vi "AdaptToInputs.vi"(0 "XRef":T8, 1 "Term Types":T5, 2 "State In":T1={"Type"=variant(bool FALSE)}) -> (14 "Reply":T3, 15 "Fatal Error Out":T2, 16 "State Out":T1={"Type"=variant(bool FALSE)})   [LabVIEW 2014, in "TagDB(dev).lvlib" / "tagDB_setValue.xnode"]
uses:
  tagDB_setValue.xnode
  <vilib>/XNodeSupport/XNodeXNodeRef.ctl
  <vilib>/XNodeSupport/XNodeTermTypeIDPairs.ctl
  <vilib>/XNodeSupport/XNodeTermTypeIDPair.ctl
  <vilib>/XNodeSupport/XNodeType.ctl
  <vilib>/XNodeSupport/XNodeString.ctl
  State.ctl
  <vilib>/XNodeSupport/XNodeStringArray.ctl
  <vilib>/XNodeSupport/XNodeErrorCluster.ctl
  <vilib>/XNodeSupport/NI_XNodeSupport.lvlib
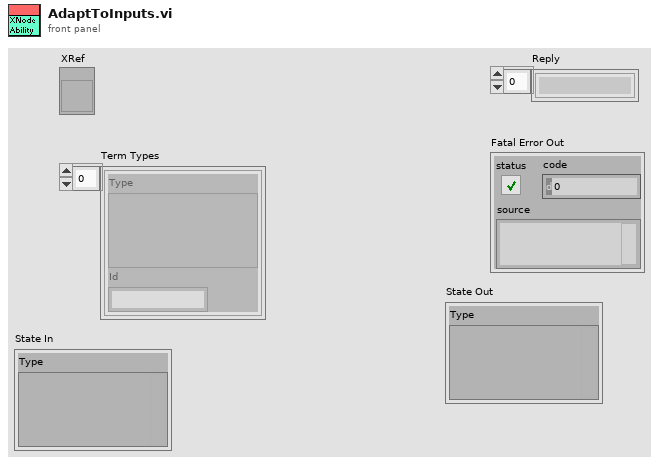
[diagram p1: front panel]
types:
  T1 = typedef "TagDB(dev).lvlib/tagDB_setValue.xnode/State.ctl" = cluster{"Type":variant}
  T2 = typedef "NI_XNodeSupport.lvlib/XNodeErrorCluster.ctl" = errorcluster
  T3 = typedef "NI_XNodeSupport.lvlib/XNodeStringArray.ctl" = T4[]
  T4 = typedef "NI_XNodeSupport.lvlib/XNodeString.ctl" = string
  T5 = typedef "NI_XNodeSupport.lvlib/XNodeTermTypeIDPairs.ctl" = T6[]
  T6 = typedef "NI_XNodeSupport.lvlib/XNodeTermTypeIDPair.ctl" = cluster{"Type":T7, "Id":T4}
  T7 = typedef "NI_XNodeSupport.lvlib/XNodeType.ctl" = variant
  T8 = typedef "NI_XNodeSupport.lvlib/XNodeXNodeRef.ctl" = refnum<vi>
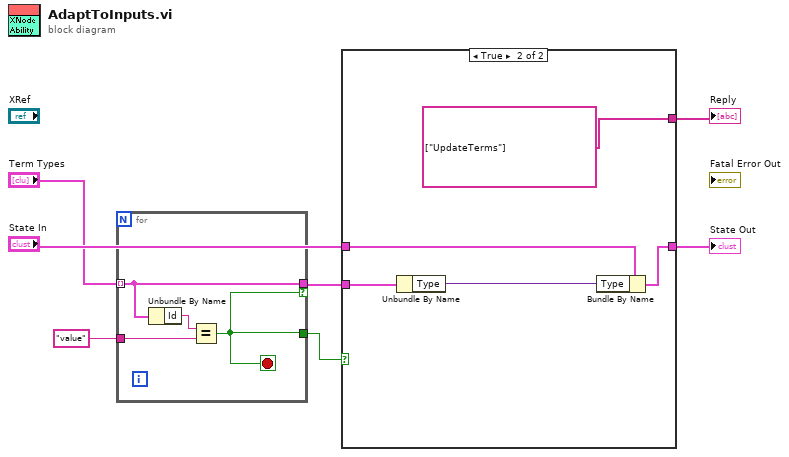
[diagram p0: block diagram]
diagram:
  n1 = for {
    tunnel: "Term Types" -> [w11] mode=indexing
    tunnel: [w11] -> w6 if=w8
    tunnel: "value" -> [w9]
    tunnel: [w8] -> w1
    stop <- w8 stop-if-true
    n2 = Unbundle By Name(w11) -> ("Id"=w10:T4)
    n3 = Equal?(x=w10, y=w9) -> (x = y?=w8:bool)
  }
  n4 = case shown="True" w1 {
    tunnel: w6 -> [_ w17]
    tunnel: [_ T3 ["UpdateTerms"] ("Reply")] -> w5
    tunnel: "State In" -> [w12 w14]
    tunnel: [w12 w13] -> w3
    frame False {
    }
    frame True {
      n5 = Unbundle By Name(w17) -> ("Type"=w16:T7)
      n6 = Bundle By Name(cluster=w14, "Type"=w16) -> (w13:T1)
    }
  }
  "Reply" <- w5
  "State Out" <- w3
